vi "Write_to_measurement.vi"() -> ()   [LabVIEW 2020]
panel:
  in  "stop":bool
  in  "Temp":dbl(slide) scale=0.0..100.0
  in  "Lim":dbl
  out "Gráfico de la Señal":dynamicdata(graph)
  out "Alarma":bool
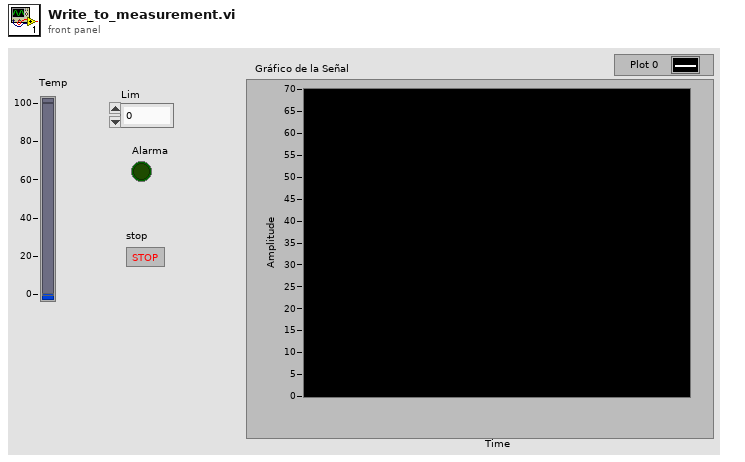
[diagram p1: front panel]
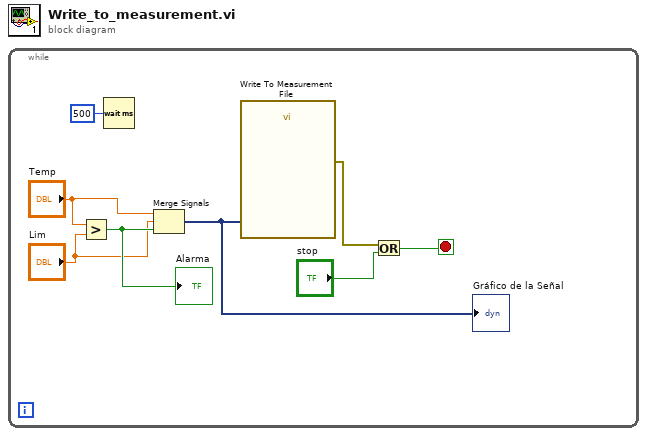
[diagram p0: block diagram]
diagram:
  n1 = while {
    stop <- w6 stop-if-true
    n2 = Greater?(x="Temp", y="Lim") -> (0:w4:bool)
    "Alarma" <- w4
    n3 = Wait (ms)(milliseconds to wait=u32 500) -> ()  [unwired: 1 out]
    n4 = Merge Signals("Temp", "Lim", w4) -> (w1:dynamicdata)
    "Gráfico de la Señal" <- w1
    n5 = call "Write To Measurement File"("Signals"=w1) -> ("error out"=w7:errorcluster)  [unwired: 16 in, 2 out]
    n6 = Or(x=w7, y="stop") -> (x .or. y?=w6:bool)
  }
